vi "DB - Split DB.Schema.Table.vi"(11 "DB.Schema.Table":string) -> (3 "DB.Schema.Table":T1)   [LabVIEW 2013]
uses:
  Controls/DB - DB.Schema.Table.ctl
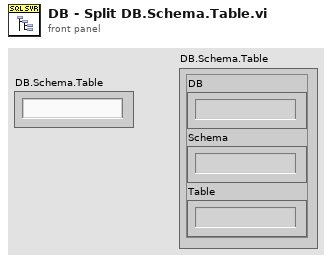
[diagram p1: front panel]
types:
  T1 = typedef "DB - DB.Schema.Table.ctl" = cluster{"DB":string, "Schema":string, "Table":string}
  T2 = cluster{"Schema":string, "DB":string, "Table":string}
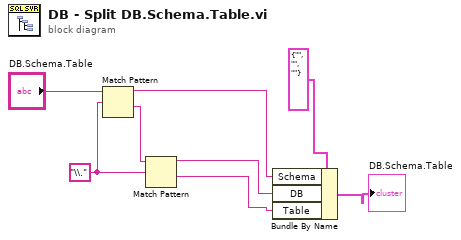
[diagram p0: block diagram]
diagram:
  w6 = "\\." ("regular expression")
  n1 = Match Pattern(string="DB.Schema.Table", regular expression=w6) -> (before substring=w3:string, after substring=w8:string)  [unwired: 1 in, 2 out]
  n2 = Match Pattern(string=w8, regular expression=w6) -> (before substring=w2:string, after substring=w1:string)  [unwired: 1 in, 2 out]
  n3 = Bundle By Name(cluster=T2 {"Schema"="", "DB"="", "Table"=""} ("DB.Schema.Table"), "Schema"=w3, "DB"=w2, "Table"=w1) -> (→"DB.Schema.Table":T2)
